vi "Estrazione Fondo - Target.vi"(11 "n-bit (2^nbit medie)":i32=8) -> ()   [LabVIEW 2014]
uses:
  <vilib>/Platform/TimedLoop/XDataNode/timing_clust.ctl
  <vilib>/Platform/TimedLoop/XDataNode/nitl_modes.ctl
  <vilib>/Platform/TimedLoop/XDataNode/wakeup.ctl
  <vilib>/rvi/Emulation/niFpgaSctlEmulationGetInTimedLoop.vi
  <vilib>/rvi/Emulation/niFpgaEmulationReportErrorSimple.vi
  <vilib>/rvi/Emulation/niFpgaGetClockAttributes.vi
  <vilib>/rvi/Emulation/niFpgaCriticalErrorInLSC.vi
  <vilib>/rvi/Memory/Memory_Emulation/nirvimemoryFastEmulation.vi
  <vilib>/rvi/Memory/Memory_Emulation/nirvimemoryEmulation.vi
  <vilib>/rvi/Emulation/niFpgaEmulationIsFPGAContextNoSignature.vi
  <vilib>/rvi/DataTransferAndStorage/Container/Common/niFpgaContainerGetUniqueNameForEmu.vi
  <vilib>/rvi/Emulation/niFpgaProcessEmulError.vi
  <vilib>/rvi/errors/nirviReportUnexpectedCaseInternalError (U32).vi
  <vilib>/rvi/errors/niFpgaSetErrorForExecOnDevCompSimple.vi
  <vilib>/rvi/eio/common/nirviEmuReportErrorAndStop.vi
  <vilib>/rvi/FIFO/Fifo_Resource/nirvififoEmulationSetSize.vi
  <vilib>/rvi/FIFO/Fifo_Resource/nirviFifoEmulationQueueMgr.vi
  <instcachedir>/0/nirviFifoEmulationQueueMgr_E5CAEC123FF24DC58D834DCA3CDAA9B5.lvgen/nirviFifoEmulationQueueMgr_E5CAEC123FF24DC58D834DCA3CDAA9B5_010.vi
  <vilib>/rvi/FIFO/Fifo_Resource/nirvififoEmulationCreateLock.vi
  <vilib>/rvi/FIFO/Fifo_Resource/nirvififoEmulationObtainLock.vi
  <vilib>/rvi/FIFO/Fifo_Resource/nirvififoEmulationReleaseLock.vi
  <vilib>/rvi/occurrence/nirviWaitOnOccurrenceBase.vi
  <vilib>/rvi/errors/nirviReportUnexpectedCaseInternalError.vi
  <vilib>/rvi/FIFO/Fifo_Resource/nirvififoEmulationDetermineInputValidOut.vi
  <vilib>/rvi/eio/common/nirviEmuTemplateMethod_errors.vi
  <vilib>/rvi/interface/RandomDataEmulation/niFpgaRandomDataHandleErrors.vi
  <vilib>/Platform/TimedLoop/XDataNode/XDataNode.xnode
  <vilib>/rvi/DataTransferAndStorage/Container/XNode/niFpgaContainer.xnode
  <vilib>/rvi/FIFO/Fifo_Resource/nirvififoEmulationRead.vi
  <vilib>/rvi/FIFO/Fifo_Resource/nirvififoEmulationWrite.vi
  <vilib>/eio/EIOMethodNode/EIOMethodNode.xnode
  <vilib>/rvi/interface/RandomDataEmulation/nirviRandomDataFpgaReadWriteTemplate.vi
  <vilib>/Platform/TimedLoop/XDataNode/XDNodeRunTimeDep.lvlib
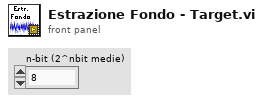
[diagram p1: front panel]
types:
  T1 = typedef "XDNodeRunTimeDep.lvlib/timing_clust.ctl" = cluster{"Expected End [f-1]":u64, "Actual End [f-1]":u64, "Finished Late? [f-1]":bool, "Expected End [i-1]":u64, "Actual End [i-1]":u64, "Finished Late? [i-1]":bool, "Expected Start [i]":u64, "Actual Start [i]":u64, "Expected Start [f]":u64, "Actual Start [f]":u64, "Source Name":string, "Structure Name":string, "Period":i64, "Deadline":i64, "Offset":i64, "Start":i64, "Priority":i32, "Timeout":i32, "Mode":T2, "Wakeup Reason":T3, "Error":errorcluster, "Source Type":string, "Secondary Source Type":string, "Global End Time":u64, "Global Start Time":u64, "Frame Duration":u64, "Iteration Duration":u64, "Assigned CPU":i32, "I/O Scan Engine Mode":u32}
  T2 = typedef "XDNodeRunTimeDep.lvlib/nitl_modes.ctl" = enum32{"No Change", "Process missed periods, maintain original phase", "Discard missed periods, maintain original phase", "Process missed periods, ignore original phase", "Discard missed periods, ignore original phase"}
  T3 = typedef "XDNodeRunTimeDep.lvlib/wakeup.ctl" = enum32{"Normal", "Aborted", "Asynchronous wakeup", "Timing source error", "Timed loop error", "Timeout"}
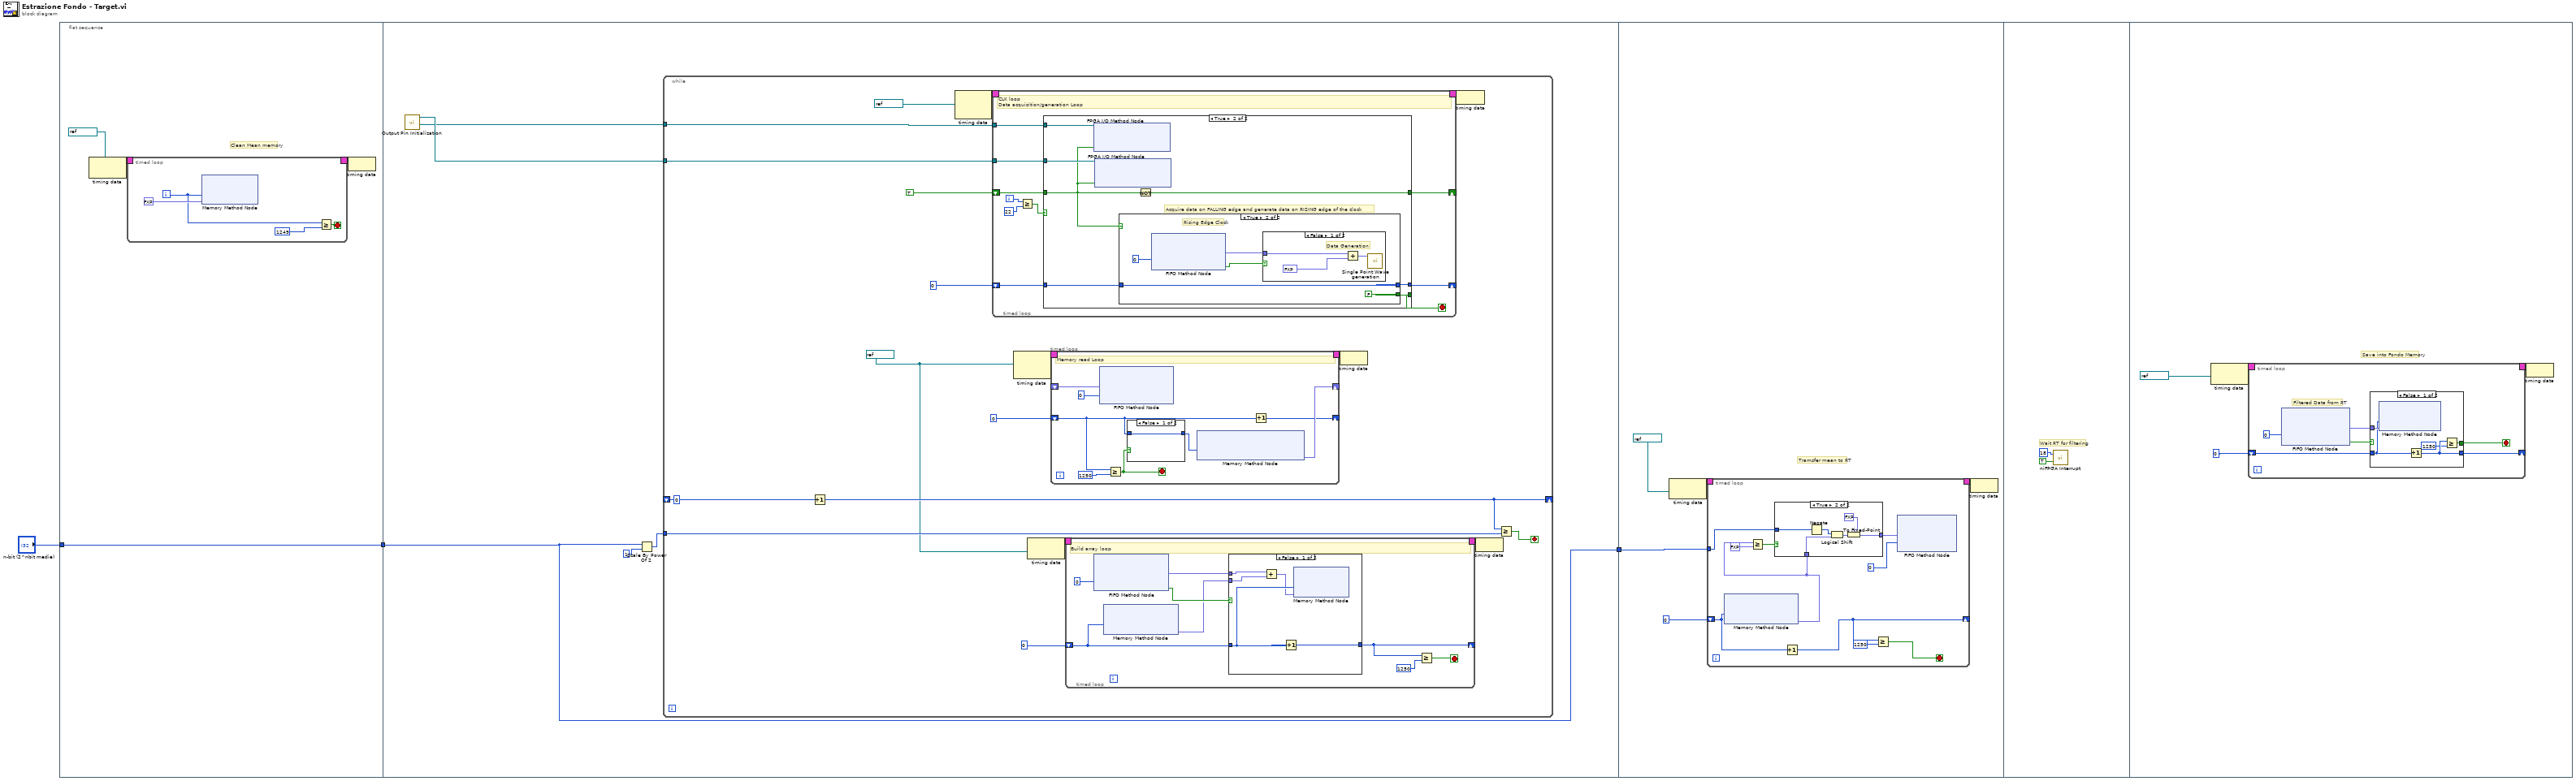
[diagram p0: block diagram]
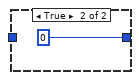
[diagram p2: hidden frame]
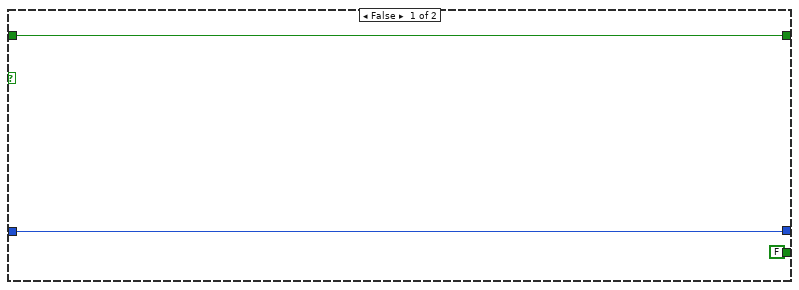
[diagram p4: hidden frame]
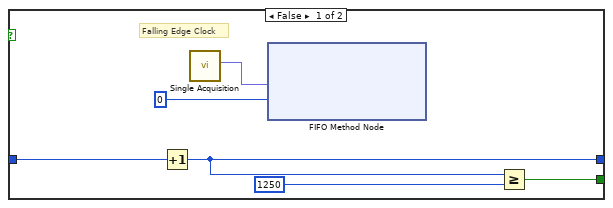
[diagram p5: hidden frame]
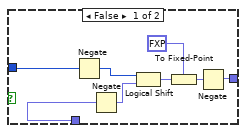
[diagram p7: hidden frame]
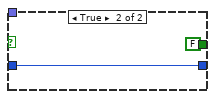
[diagram p8: hidden frame]
diagram:
  n1 = flat-sequence {
    tunnel: [w5] -> w2
    tunnel: "n-bit (2^nbit medie)" -> [w5]
    tunnel: [w18] -> w3
    tunnel: w2 -> [w18]
    tunnel: w3 -> [w119]
    frame #0 {
      # "Clean Mean memory"
      n2 = node-c288(refnum<k21> "30MHz" ("Source Name")) -> (w7:T1)
      n3 = timed-loop {
        timing: w7 -> [_]
        timing-out: [_] -> w6
        i -> [w10]
        stop <- w9 stop-if-true
        n4 = xnode ("Memory Method Node")("Address"=w10, "Data"=fxp<+/-,24,24> 0.0) -> ()  [unwired: 1 in, 1 out]
        n5 = Greater Or Equal?(x=w10, y=1249) -> (x >= y?=w9:bool)
      }
      n6 = node-c288(w6) -> ()
    }
    frame #1 {
      n7 = call "Output Pin Initialization.vi"() -> ("I/O Out Clock DAC (pin16)"=w22:refnum<k21>, "I/O Out Clock ADC (pin17)"=w23:refnum<k21>)  [unwired: 8 in, 1 out]
      n8 = Scale By Power Of 2(n=w18, x=1) -> (x*2^n=w19:i32)
      n9 = while {
        shift-right: [w39] -> _
        shift-left: 0 -> [w40]
        tunnel: w23 -> [w36]
        tunnel: w22 -> [w35]
        tunnel: w19 -> [w26]
        stop <- w41 stop-if-true
        w24 = refnum<k21> "30MHz" ("Source Name")
        n10 = Increment(x=w40) -> (x+1=w39:i32)
        n11 = node-c288(refnum<k21> "60MHz" ("Source Name")) -> (w38:T1)  [unwired: 1 in]
        n12 = timed-loop {
          timing: w38 -> [_]
          timing-out: [_] -> w37
          shift-right: [w86] -> _
          shift-left: TRUE -> [w84]
          tunnel: w35 -> [w87]
          tunnel: w36 -> [w85]
          shift-right: [w82] -> _
          shift-left: 0 -> [w83]
          i -> [w81]
          stop <- w79 stop-if-true
          # "CLK loop\nData acquisition/generation Loop"
          n13 = Greater Or Equal?(x=w81, y=22) -> (x >= y?=w80:bool)
          n14 = case shown="True" w80 {
            tunnel: w87 -> [_ w97]
            tunnel: [w89 w96] -> w86
            tunnel: w85 -> [_ w95]
            tunnel: w84 -> [w89 w91]
            tunnel: w83 -> [w90 w94]
            tunnel: [FALSE w93] -> w79
            tunnel: [w90 w92] -> w82
            frame False {
            }
            frame True {
              # "Acquire data on FALLING edge and generate data on RISING edge of the clock"
              n15 = xnode "FPGA I/O Method Node"("FPGA I/O In"=w97, "Data"=w91) -> ()  [unwired: 1 out]
              n16 = xnode "FPGA I/O Method Node"("FPGA I/O In"=w95, "Data"=w91) -> ()  [unwired: 1 out]
              n17 = case shown="True" w91 {
                tunnel: w94 -> [w103 w105]
                tunnel: [w101 FALSE] -> w93
                tunnel: [w98 w105] -> w92
                frame False {
                  # "Falling Edge Clock"
                  n18 = Increment(x=w103) -> (x+1=w98:i32)
                  n19 = call "Single Acquisition.vi"() -> ("Out"=w100:fxp<+/-,12,12>)  [unwired: 10 in, 1 out]
                  n20 = xnode ("FIFO Method Node")("Element"=w100, "Timeout"=0) -> ()  [unwired: 1 in, 2 out]
                  n21 = Greater Or Equal?(x=w98, y=1250) -> (x >= y?=w101:bool)
                }
                frame True {
                  # "Rising Edge Clock"
                  n22 = xnode ("FIFO Method Node")("Timeout"=0) -> ("Element"=w106:fxp<+/-,12,12>, "Timed Out?"=w107:bool)  [unwired: 1 in, 1 out]
                  n23 = case shown="False" w107 {
                    tunnel: w106 -> [w111 _]
                    frame False {
                      # "Data Generation"
                      n24 = Add(x=w111, y=fxp<+,12,12> 2048.0) -> (x+y=w109:fxp<+/-,14,14>)
                      n25 = call "Single Point Wave generation.vi"("Data To Write"=w109) -> ()  [unwired: 10 in, 1 out]
                    }
                    frame True {
                      # "FPGA memory slow"
                    }
                  }
                }
              }
              n26 = Not(x=w91) -> (.not. x?=w96:bool)
            }
          }
        }
        n27 = node-c288(w24) -> (w29:T1)  [unwired: 1 in]
        n28 = node-c288(w24) -> (w32:T1)
        n29 = timed-loop {
          timing: w29 -> [_]
          timing-out: [_] -> w28
          shift-right: [w45] -> _
          shift-left: u32 0 -> [w43]
          shift-right: [w47] -> _
          shift-left: _ -> [w46]
          stop <- w44 stop-if-true
          # "Memory read Loop"
          n30 = xnode ("FIFO Method Node")("Element"=w46, "Timeout"=0) -> ()  [unwired: 1 in, 2 out]
          n31 = Greater Or Equal?(x=w43, y=u32 1250) -> (x >= y?=w44:bool)
          n32 = case shown="False" w44 {
            tunnel: w43 -> [w50 _]
            tunnel: [w50 u32 0] -> w42
            frame False {
            }
            frame True {
            }
          }
          n33 = xnode ("Memory Method Node")("Address"=w42) -> ("Data"=w47:fxp<+/-,12,12>)  [unwired: 1 in, 1 out]
          n34 = Increment(x=w43) -> (x+1=w45:u32)
        }
        n35 = timed-loop {
          timing: w32 -> [_]
          timing-out: [_] -> w31
          shift-right: [w63] -> _
          shift-left: u32 0 ("Address") -> [w59]
          stop <- w61 stop-if-true
          # "Build array loop"
          n36 = xnode ("FIFO Method Node")("Timeout"=0) -> ("Element"=w64:fxp<+/-,12,12>, "Timed Out?"=w62:bool)  [unwired: 1 in, 1 out]
          n37 = xnode ("Memory Method Node")("Address"=w59) -> ("Data"=w60:fxp<+/-,24,24>)  [unwired: 1 in, 1 out]
          n38 = case shown="False" w62 {
            tunnel: w64 -> [w68 _]
            tunnel: w59 -> [w69 w71]
            tunnel: [w70 w71] -> w63
            tunnel: w60 -> [w67 _]
            frame False {
              n39 = Add(x=w68, y=w67) -> (x+y=w66:fxp<+/-,24,24>)
              n40 = Increment(x=w69) -> (x+1=w70:u32)
              n41 = xnode ("Memory Method Node")("Address"=w69, "Data"=w66) -> ()  [unwired: 1 in, 1 out]
            }
            frame True {
            }
          }
          n42 = Greater Or Equal?(x=w63, y=u32 1250) -> (x >= y?=w61:bool)
        }
        n43 = node-c288(w28) -> ()
        n44 = node-c288(w37) -> ()
        n45 = node-c288(w31) -> ()
        n46 = Greater Or Equal?(x=w39, y=w26) -> (x >= y?=w41:bool)
      }
    }
    frame #2 {
      # "Tramsfer mean to RT"
      n47 = node-c288(refnum<k21> "30MHz" ("Source Name")) -> (w122:T1)
      n48 = timed-loop {
        tunnel: w119 -> [w126]
        timing: w122 -> [_]
        timing-out: [_] -> w121
        shift-right: [w130] -> _
        shift-left: u32 0 ("Address") -> [w131]
        stop <- w129 stop-if-true
        n49 = xnode ("Memory Method Node")("Address"=w131) -> ("Data"=w125:fxp<+/-,24,24>)  [unwired: 1 in, 1 out]
        n50 = Greater Or Equal?(x=w125, y=fxp<+/-,24,24> 0.0) -> (x >= y?=w124:bool)
        n51 = case shown="True" w124 {
          tunnel: w125 -> [w136 w146]
          tunnel: [w133 w144] -> w127
          tunnel: w126 -> [w137 w142]
          frame False {
            n52 = Negate(x=w137) -> (-x=w140:i32)
            n53 = Negate(x=w136) -> (-x=w135:fxp<+/-,24,24>)
            n54 = Logical Shift(y=w140, x=w135) -> (x << y=w138:fxp<+/-,24,24>)
            n55 = To Fixed-Point(fixed-point type=fxp<+/-,12,12> 0.0 ("Element"), number=w138) -> (fixed-point=w134:fxp<+/-,12,12>)
            n56 = Negate(x=w134) -> (-x=w133:fxp<+/-,12,12>)
          }
          frame True {
            n57 = Negate(x=w142) -> (-x=w141:i32)
            n58 = Logical Shift(y=w141, x=w146) -> (x << y=w145:fxp<+/-,24,24>)
            n59 = To Fixed-Point(fixed-point type=fxp<+/-,12,12> 0.0 ("Element"), number=w145) -> (fixed-point=w144:fxp<+/-,12,12>)
          }
        }
        n60 = Increment(x=w131) -> (x+1=w130:u32)
        n61 = Greater Or Equal?(x=w130, y=u32 1250) -> (x >= y?=w129:bool)
        n62 = xnode ("FIFO Method Node")("Element"=w127, "Timeout"=0) -> ()  [unwired: 1 in, 2 out]
      }
      n63 = node-c288(w121) -> ()
    }
    frame #3 {
      # "Wait RT for filtering"
      n64 = call <vilib>:"niFPGA Interrupt.vi"("Wait Until Cleared (F)"=TRUE, "IRQ Number (0)"=u8 18) -> ()  [unwired: 1 in]
    }
    frame #4 {
      # "Save into Fondo Memory"
      n65 = node-c288(refnum<k21> "30MHz" ("Source Name")) -> (w158:T1)
      n66 = timed-loop {
        timing: w158 -> [_]
        timing-out: [_] -> w157
        shift-right: [w160] -> _
        shift-left: u32 0 ("Address") -> [w162]
        stop <- w161 stop-if-true
        # "Filtered Data from RT"
        n67 = xnode ("FIFO Method Node")("Timeout"=0) -> ("Element"=w163:fxp<+/-,12,12>, "Timed Out?"=w159:bool)  [unwired: 1 in, 1 out]
        n68 = case shown="False" w159 {
          tunnel: w163 -> [w169 _]
          tunnel: w162 -> [w168 w171]
          tunnel: [w167 FALSE] -> w161
          tunnel: [w166 w171] -> w160
          frame False {
            n69 = xnode ("Memory Method Node")("Address"=w168, "Data"=w169) -> ()  [unwired: 1 in, 1 out]
            n70 = Increment(x=w168) -> (x+1=w166:u32)
            n71 = Greater Or Equal?(x=w166, y=u32 1250) -> (x >= y?=w167:bool)
          }
          frame True {
          }
        }
      }
      n72 = node-c288(w157) -> ()
    }
  }
